vi "ma_put 1.vi"(8 "Error":errorcluster, 11 "KNR in":T1) -> (0 "error out 4":errorcluster caption="error out", 2 "最終堆疊版":bool[][](array[boolean]), 3 "KNR out":T1, 5 "x1":dbl)   [LabVIEW 2013]
uses:
  <userlib>/_FPGA Interface Advanced Tools/FPGA Interface Base/FPGA Interface Base.lvclass
  <userlib>/KNR OS 3.0 LabVIEW Toolkit/Type Definition/Resource.ctl
  <userlib>/KNR OS 3.0 LabVIEW Toolkit/Type Definition/KNR3 Reference.ctl
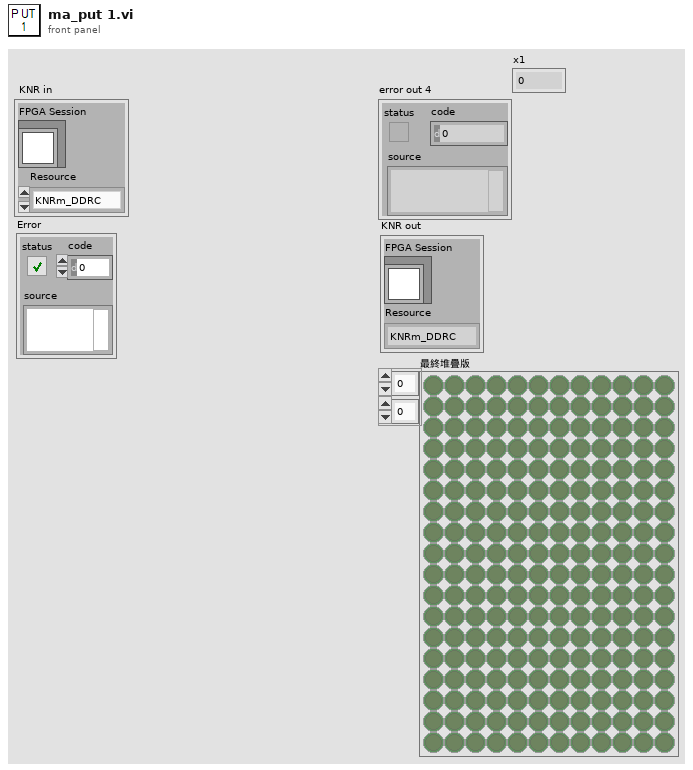
[diagram p1: front panel]
types:
  T1 = typedef "KNR3 Reference.ctl" = cluster{"FPGA Session":refnum<class "FPGA Interface Base.lvclass">, "Resource":T2}
  T2 = typedef "Resource.ctl" = enum16{"KNRm_DDRC", "KNRm_DDDD", "KNRm_DDDR", "KNRm_DDDC", "KNR"}
  T3 = cluster{"Position":cluster{"X":sgl, "Y":sgl}, "Radius":dbl, "Score":dbl}[]
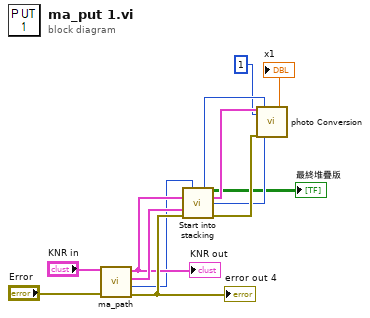
[diagram p0: block diagram]
diagram:
  n1 = call "ma_path.vi"("Error"="Error", "KNR in"="KNR in") -> ("error out 4"=w12:errorcluster, "Number of Matches (Shape Detection 1)"=w10:i32, "Circles (Shape Detection 1)"=w13:T3, "KNR out"=w11:T1)  [unwired: 4 in, 2 out]
  "error out 4" <- w12
  "KNR out" <- w11
  n2 = call "Start into stacking.vi"("ふ计"=w10, "KNR in"=w11, "Circles (Shape Detection 1) 2"=w13, "Error"=w12) -> ("X"=w4:i32, "最終堆疊版"=→"最終堆疊版":bool[][], "KNR out"=w7:T1, "底盤T數"=w5:i32, "error out"=w6:errorcluster)  [unwired: 2 in, 5 out]
  n3 = call "photo Conversion.vi"("KNR in"=w7, "順序"=1, "error in"=w6, "x1"=w4, "t1"=w5) -> ("x"=→"x1":dbl)  [unwired: 12 in, 2 out]
